vi "HandleInput.vi"(8 "Variant":variant, 9 "Type":i32, 10 "Messge in":refnum<class "BaseMessage.lvclass">, 11 "BaseDriver in":refnum<class "BaseDriver.lvclass">) -> (1 "Send message?":bool, 2 "Messages out":refnum<class "BaseMessage.lvclass">[](array[class]), 3 "BaseDriver out":refnum<class "BaseDriver.lvclass">)   [LabVIEW 2018, in "BaseDriver.lvclass"]
doc: "Callback for any messages from the calling application handled by the driver. Overload to do any special handling"
uses:
  BaseDriver.lvclass
  Message/BaseMessage/BaseMessage.lvclass
  BaseDriver.lvclass/BaseDriver.ctl
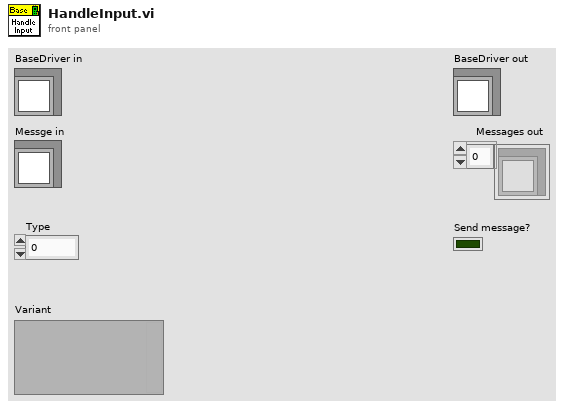
[diagram p1: front panel]
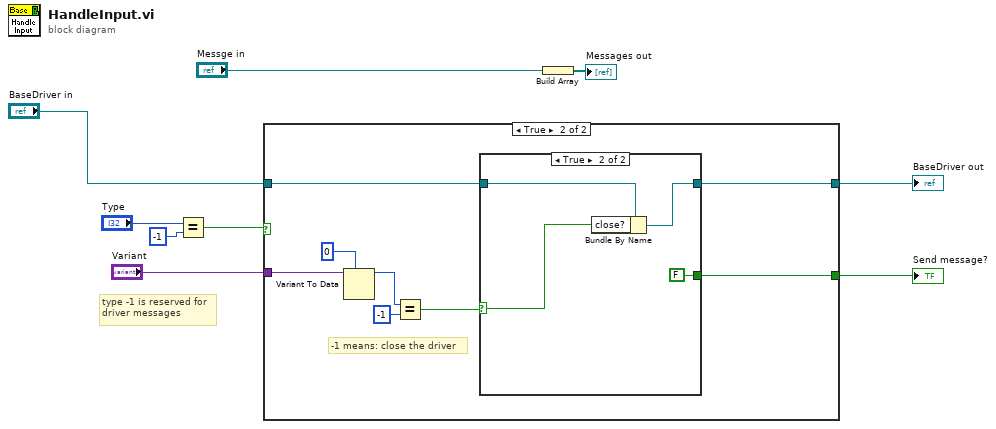
[diagram p0: block diagram]
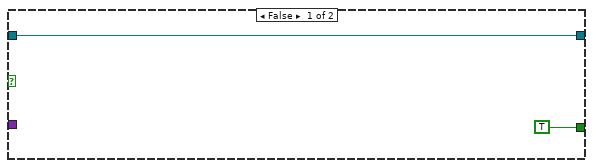
[diagram p2: hidden frame]
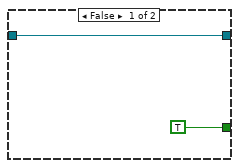
[diagram p3: hidden frame]
diagram:
  # "type -1 is reserved for\ndriver messages"
  n1 = Equal?(x="Type", y=-1) -> (x = y?=w7:bool)
  n2 = case shown="True" w7 {
    tunnel: "Variant" -> [_ w19]
    tunnel: "BaseDriver in" -> [w10 w15]
    tunnel: [w10 w14] -> w4
    tunnel: [TRUE ("Send message?") w12] -> w3
    frame False {
    }
    frame True {
      # "-1 means: close the driver"
      n3 = Variant To Data(type=0 ("y"), Variant=w19) -> (data=w16:i32)  [unwired: 1 in, 1 out]
      n4 = Equal?(x=w16, y=-1) -> (x = y?=w13:bool)
      n5 = case shown="True" w13 {
        selector: w13 -> [_ w22]
        tunnel: w15 -> [w21 w25]
        tunnel: [w21 w24] -> w14
        tunnel: [TRUE ("Send message?") FALSE ("Send message?")] -> w12
        frame False {
        }
        frame True {
          n6 = Bundle By Name(cluster=w25, "close?"=w22) -> (w24:refnum<class "BaseDriver.lvclass">)
        }
      }
    }
  }
  "BaseDriver out" <- w4
  "Send message?" <- w3
  n7 = Build Array("Messge in") -> (→"Messages out":refnum<class "BaseMessage.lvclass">[])
